vi "Periodic Tasks.vi"(8 "error in":errorcluster) -> ()   [LabVIEW 2019]
doc: "This VI runs in parallel to other tasks. It can contain as many user-defined periodic loops as you need. These can carry out PID or other sorts of timed response."
uses:
  <vilib>/Rock Robotics/WPI/DriverStation/WPI_DriverStationRobotMode2.ctl
  <vilib>/Rock Robotics/WPI/Utilities/WPI_GetSetVariantRefNum.vi
  Robot Global Data.vi
  <vilib>/Rock Robotics/WPI/RobotDrive/WPI_RobotDriveArcadeDrive_Standard(NoSaturation).vi
  <vilib>/Rock Robotics/Network Tables/NT Write Numeric Array.vi
  <vilib>/Rock Robotics/Network Tables/NT Write Number.vi
  <vilib>/Rock Robotics/Network Tables/NT Write String.vi
panel:
  in  "Yellow":cluster{"R":dbl, "G":dbl, "B":dbl}
  in  "Blue":cluster{"R":dbl, "G":dbl, "B":dbl}
  in  "Green":cluster{"R":dbl, "G":dbl, "B":dbl}
  in  "Red":cluster{"R":dbl, "G":dbl, "B":dbl}
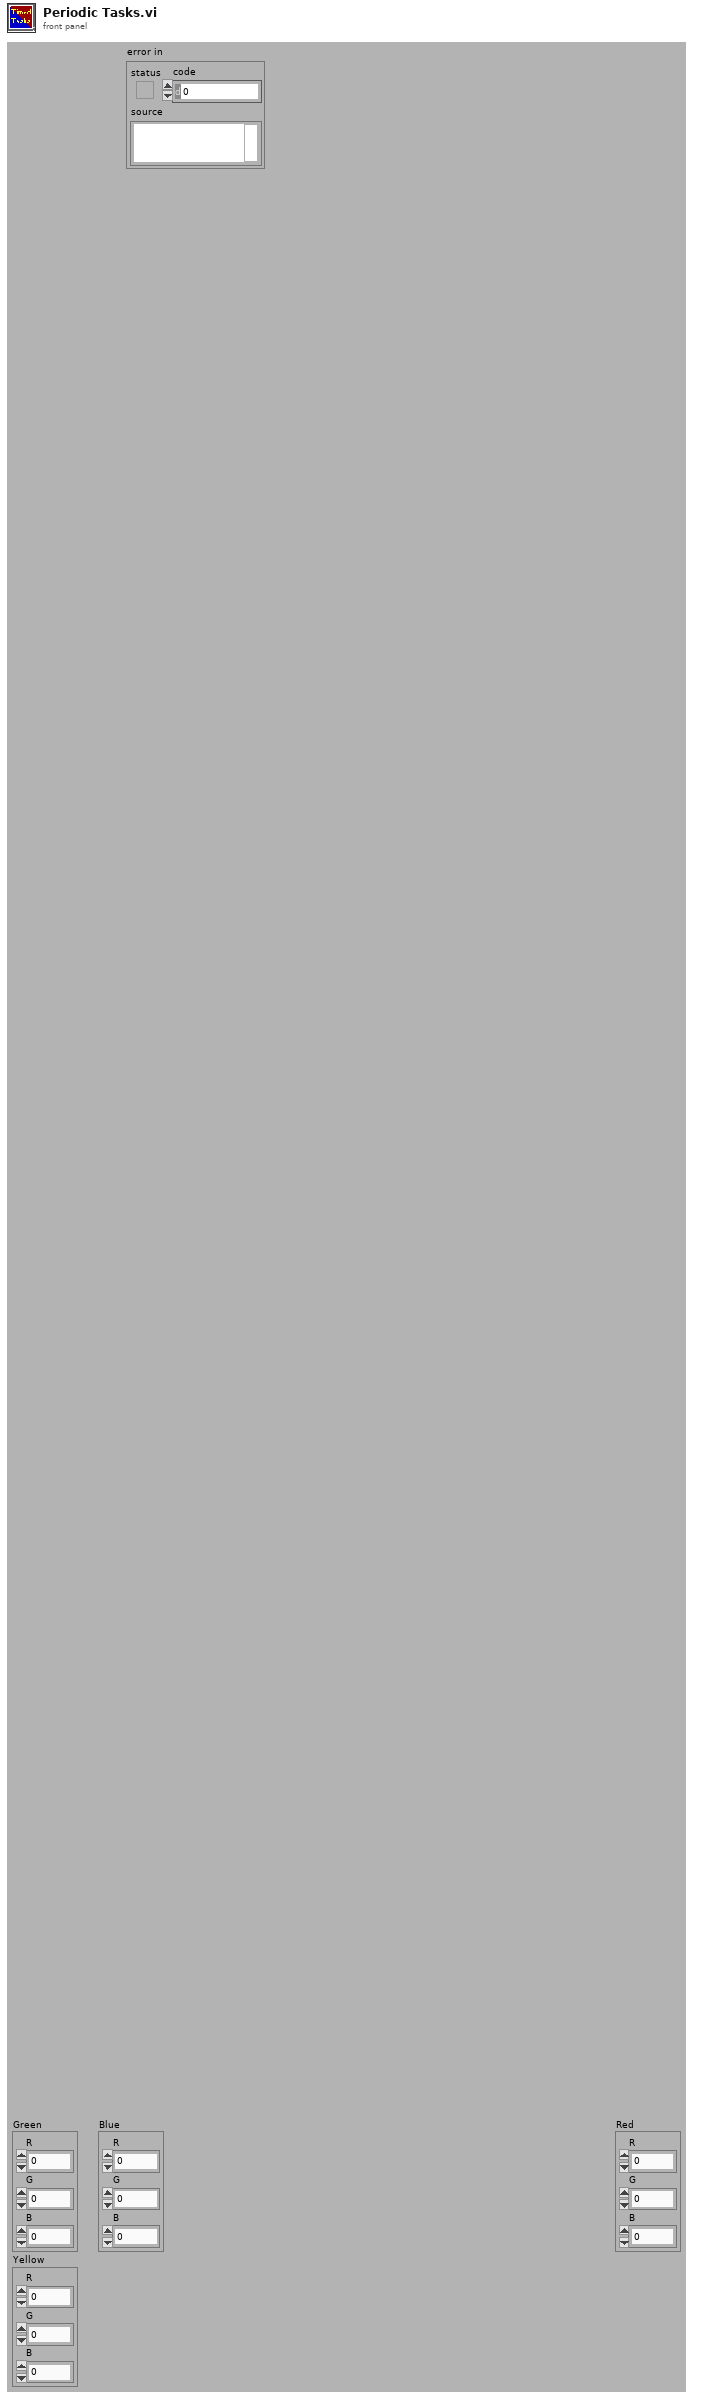
[diagram p1: front panel]
types:
  T1 = typedef "WPI_RobotDriveDevRef.ctl" = cluster{"DevStatus":errorcluster, "Motors[]":T2[], "Square Inputs":bool, "Max Output":dbl}
  T2 = typedef "WPI_MotorControlDeviceRef.ctl" = cluster{"DeviceStatus":errorcluster, "Type":T3, "PWM":cluster{"PWM Channel":T4, "DeadBand":T5}, "CAN":cluster{"Device Number":u8, "SetOutput VI Ref":variant, "GetOutput VI Ref":variant, "Enable VI Ref":variant, "Disable VI Ref":variant, "Data":variant}, "Invert":bool, "DIO PWM":cluster{"PWM \"Enable\" Channel":T4, "DIOChannel":T6, "PWM Rate":dbl}}
  T3 = typedef "WPI_MotorControlType.ctl" = enum16{"PWM", "CAN", "DIO PWM"}
  T4 = typedef "FPGA_DIOPWMChannel.ctl" = enum8{"PWM 0", "PWM 1", "PWM 2", "PWM 3", "PWM 4", "PWM 5", "PWM 6", "PWM 7", "PWM 8", "PWM 9", "PWM MXP 0", "PWM MXP 1", "PWM MXP 2", "PWM MXP 3", "PWM MXP 4", "PWM MXP 5", "PWM MXP 6", "PWM MXP 7", "PWM MXP 8", "PWM MXP 9", "Invalid"}
  T5 = typedef "WPI_PWMDeadband.ctl" = cluster{"Name":string, "maxPositivePwm":i32, "minPositivePwm":i32, "centerPwm":i32, "maxNegativePwm":i32, "minNegativePwm":i32, "angularRange":u16}
  T6 = typedef "FPGA_DIOChannel.ctl" = enum8{"DIO 0", "DIO 1", "DIO 2", "DIO 3", "DIO 4", "DIO 5", "DIO 6", "DIO 7", "DIO 8", "DIO 9", "DIO MXP 0", "DIO MXP 1", "DIO MXP 2", "DIO MXP 3", "DIO MXP 4", "DIO MXP 5", "DIO MXP 6", "DIO MXP 7", "DIO MXP 8", "DIO MXP 9", "DIO MXP 10", "DIO MXP 11", "DIO MXP 12", "DIO MXP 13", "DIO MXP 14", "DIO MXP 15", "SPI Port CS1", "SPI Port CS2", "SPI Port CS3", "SPI Port MISO", "SPI Port MOSI", "Invalid"}
  T7 = typedef "WPI_JoystickDevRef.ctl" = cluster{"Device":T8}
  T8 = typedef "WPI_JoystickDeviceEnum.ctl" = enum16{"USB 0", "USB 1", "USB 2", "USB 3", "USB 4", "USB 5"}
  T9 = cluster{"JoystickDevRef":T7, "RobotDriveDevRef":T1}
  T10 = typedef "WPI_DriverStationRobotMode2.ctl" = enum16{"Autonomous Disabled", "Autonomous Enabled", "Teleop Disabled", "Teleop Enabled", "Disconnected", "Finish", "Test Disabled", "Test Enabled", "Emergency Stopped"}
  T11 = typedef "Color Sensor V3 DevRef.ctl" = cluster{"I2CDevRef":T12}
  T12 = typedef "WPI_I2CDevRef.ctl" = cluster{"DevStatus":errorcluster, "Device Address":u8, "Handle":i32, "I2C Bus":T13}
  T13 = typedef "i2c_bus.ctl" = enum16{"I2C On-Board", "I2C MXP", "Invalid"}
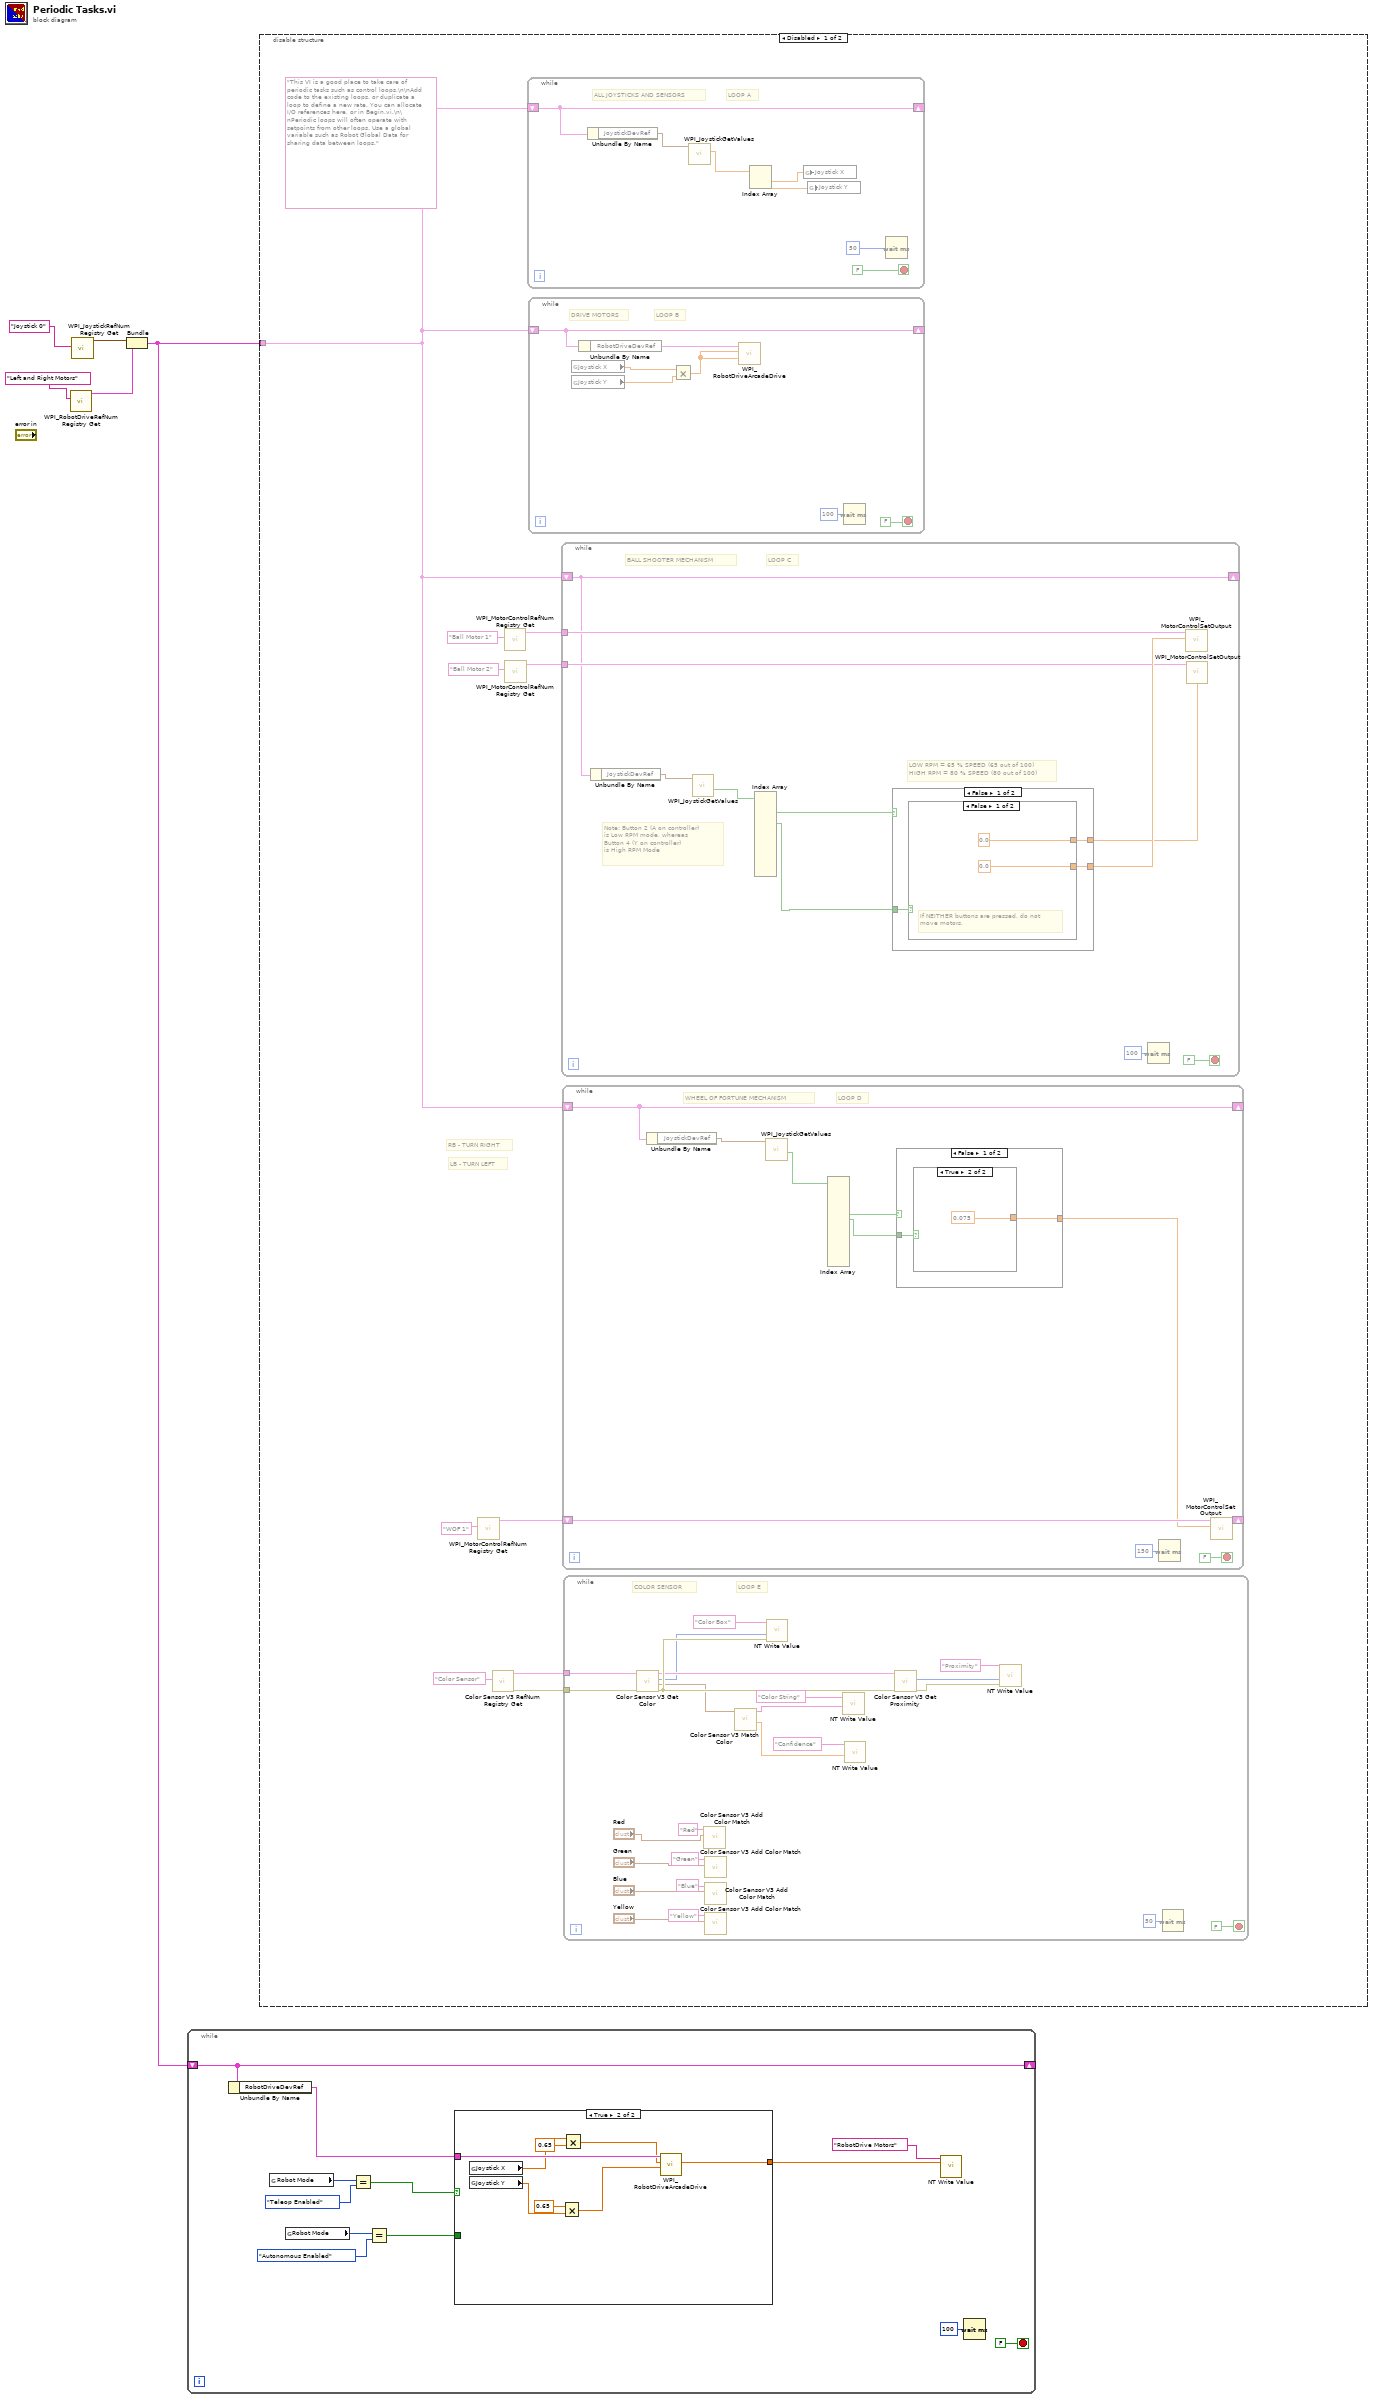
[diagram p0: block diagram]
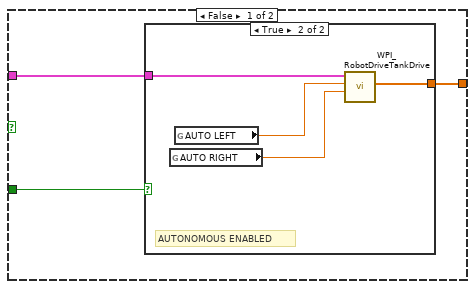
[diagram p2: hidden frame]
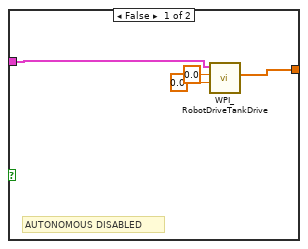
[diagram p3: hidden frame]
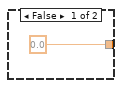
[diagram p4: hidden frame]
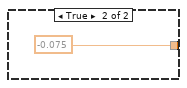
[diagram p5: hidden frame]
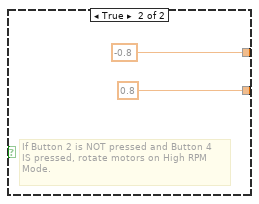
[diagram p6: hidden frame]
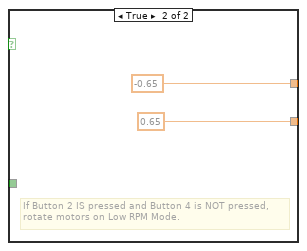
[diagram p7: hidden frame]
diagram:
  n1 = call <vilib>:"WPI_RobotDriveRefNum Registry Get.vi"("refnum name"="Left and Right Motors") -> ("RobotDriveDevRef"=w5:T1)  [unwired: 1 in, 9 out]
  n2 = call <vilib>:"WPI_JoystickRefNum Registry Get.vi"("refnum name"="Joystick 0") -> ("JoystickDevRef"=w4:T7)  [unwired: 1 in, 9 out]
  n3 = Bundle("JoystickDevRef"=w4, "RobotDriveDevRef"=w5) -> (w1:T9)  [unwired: 1 out]
  n4 = while {
    shift-right: [w17] -> _
    shift-left: w1 -> [w17]
    stop <- FALSE stop-if-true
    n5 = Unbundle By Name(w17) -> ("RobotDriveDevRef"=w12:T1)
    n6 = global read "Robot Global Data.vi" "Robot Mode"() -> (w10:T10)
    n7 = global read "Robot Global Data.vi" "Robot Mode"() -> (w8:T10)
    n8 = Equal?(x=w10, y=WPI_DriverStationRobotMode2."Teleop Enabled") -> (x = y?=w11:bool)
    n9 = Equal?(x=w8, y=WPI_DriverStationRobotMode2."Autonomous Enabled") -> (x = y?=w6:bool)
    n10 = case shown="True" w11 {
      tunnel: [w20 w35] -> w13
      tunnel: w12 -> [w19 w36]
      tunnel: w6 -> [w18 _]
      frame False {
        n11 = case shown="True" w18 {
          tunnel: [w24 w28] -> w20
          tunnel: w19 -> [w21 w26]
          frame False {
            # "AUTONOMOUS DISABLED"
            n12 = call <vilib>:"WPI_RobotDriveTankDrive.vi"("Right axis value"=0.0, "Left axis value"=0.0, "RobotDriveDevRef"=w21) -> ("Motor Values"=w24:dbl[])  [unwired: 6 in, 2 out]
          }
          frame True {
            # "AUTONOMOUS ENABLED"
            n13 = global read "Robot Global Data.vi" "AUTO RIGHT"() -> (w25:dbl)
            n14 = global read "Robot Global Data.vi" "AUTO LEFT"() -> (w27:dbl)
            n15 = call <vilib>:"WPI_RobotDriveTankDrive.vi"("Right axis value"=w25, "Left axis value"=w27, "RobotDriveDevRef"=w26) -> ("Motor Values"=w28:dbl[])  [unwired: 6 in, 2 out]
          }
        }
      }
      frame True {
        n16 = global read "Robot Global Data.vi" "Joystick X"() -> (w34:dbl)
        n17 = global read "Robot Global Data.vi" "Joystick Y"() -> (w33:dbl)
        n18 = Multiply(x=0.65, y=w33) -> (x*y=w29:dbl)
        n19 = Multiply(x=w34, y=0.65) -> (x*y=w30:dbl)
        n20 = call-poly <vilib>:"WPI_RobotDriveArcadeDrive.vi"("Y axis value"=w29, "X axis value"=w30, "RobotDriveDevRef"=w36) -> ("Motor Values"=w35:dbl[])  [unwired: 6 in, 2 out]
      }
    }
    n21 = call-poly <vilib>:"NT Write Value.vi"("Numeric Array"=w13, "Name"="RobotDrive Motors") -> ()  [unwired: 9 in, 1 out]
    n22 = Wait (ms)(milliseconds to wait=u32 100) -> ()  [unwired: 1 out]
  }
  n23 = disable-structure shown="Disabled" {
    disable-tunnel: w1 -> [w37 _]
    frame Disabled {
      (unwired) "This VI is a good place to take care of periodic tasks such as control loops.\n\nAdd code to the existing loops, or duplicate a loop to define a new rate. You can allocate I/O references here, or in Begin.vi.\n\nPeriodic loops will often operate with setpoints from other loops. Use a global variable such as Robot Global Data for sharing data between loops."
      # "LB - TURN LEFT"
      # "RB - TURN RIGHT"
      n24 = call <vilib>:"WPI_MotorControlRefNum Registry Get.vi"("refnum name"="WOF 1") -> ("MotorControlDevRef"=w41:T2)  [unwired: 9 in, 1 out]
      n25 = call <vilib>:"Color Sensor V3 RefNum Registry Get.vi"("refnum name"="Color Sensor") -> ("error out"=w38:errorcluster, "ColorSensorDevRef"=w40:T11)  [unwired: 9 in]
      n26 = call <vilib>:"WPI_MotorControlRefNum Registry Get.vi"("refnum name"="Ball Motor 1") -> ("MotorControlDevRef"=w44:T2)  [unwired: 9 in, 1 out]
      n27 = call <vilib>:"WPI_MotorControlRefNum Registry Get.vi"("refnum name"="Ball Motor 2") -> ("MotorControlDevRef"=w43:T2)  [unwired: 9 in, 1 out]
      n28 = while {
        shift-right: [w118] -> _
        shift-left: w37 -> [w118]
        stop <- FALSE stop-if-true
        # "LOOP A"
        # "ALL JOYSTICKS AND SENSORS"
        n29 = Unbundle By Name(w118) -> ("JoystickDevRef"=w117:T7)
        n30 = call <vilib>:"WPI_JoystickGetValues.vi"("JoystickDevRef"=w117) -> ("Axes"=w116:dbl[])  [unwired: 6 in, 4 out]
        n31 = Index Array(array=w116) -> (element #1=w114:dbl, element #2=w115:dbl)  [unwired: 2 in]
        n32 = global write "Robot Global Data.vi" "Joystick X"(w114) -> ()
        n33 = global write "Robot Global Data.vi" "Joystick Y"(w115) -> ()
        n34 = Wait (ms)(milliseconds to wait=u32 50) -> ()  [unwired: 1 out]
      }
      n35 = while {
        shift-right: [w110] -> _
        shift-left: w37 -> [w110]
        stop <- FALSE stop-if-true
        # "LOOP B"
        # "DRIVE MOTORS"
        n36 = global read "Robot Global Data.vi" "Joystick X"() -> (w106:dbl)
        n37 = global read "Robot Global Data.vi" "Joystick Y"() -> (w107:dbl)
        n38 = Unbundle By Name(w110) -> ("RobotDriveDevRef"=w109:T1)
        n39 = Multiply(x=w106, y=w107) -> (x*y=w108:dbl)
        n40 = call-poly <vilib>:"WPI_RobotDriveArcadeDrive.vi"("Y axis value"=w108, "X axis value"=w108, "RobotDriveDevRef"=w109) -> ()  [unwired: 6 in, 3 out]
        n41 = Wait (ms)(milliseconds to wait=u32 100) -> ()  [unwired: 1 out]
      }
      n42 = while {
        shift-right: [w90] -> _
        shift-left: w37 -> [w90]
        tunnel: w44 -> [w94]
        tunnel: w43 -> [w91]
        stop <- FALSE stop-if-true
        # "LOW RPM = 65 % SPEED (65 out of 100)\nHIGH RPM = 80 % SPEED (80 out of 100)"
        # "LOOP C"
        # "Note: Button 2 (A on controller) \nis Low RPM mode, whereas \nButton 4 (Y on controller)\nis High RPM Mode"
        # "BALL SHOOTER MECHANISM"
        n43 = Unbundle By Name(w90) -> ("JoystickDevRef"=w89:T7)
        n44 = call <vilib>:"WPI_JoystickGetValues.vi"("JoystickDevRef"=w89) -> ("Buttons"=w88:bool[])  [unwired: 6 in, 4 out]
        n45 = Index Array(array=w88) -> (element #2=w86:bool, element #4=w87:bool)  [unwired: 13 in, 11 out]
        n46 = case shown="False" w86 {
          tunnel: [w99 0.65 ("Output")] -> w93
          tunnel: [w98 -0.65 ("Output")] -> w92
          tunnel: w87 -> [w97 _]
          frame False {
            n47 = case shown="False" w97 {
              tunnel: [0.0 ("Output") 0.8 ("Output")] -> w99
              tunnel: [0.0 ("Output") -0.8 ("Output")] -> w98
              frame False {
                # "If NEITHER buttons are pressed, do not\nmove motors."
              }
              frame True {
                # "If Button 2 is NOT pressed and Button 4\nIS pressed, rotate motors on High RPM\nMode."
              }
            }
          }
          frame True {
            # "If Button 2 IS pressed and Button 4 is NOT pressed,\nrotate motors on Low RPM Mode."
          }
        }
        n48 = Wait (ms)(milliseconds to wait=u32 100) -> ()  [unwired: 1 out]
        n49 = call <vilib>:"WPI_MotorControlSetOutput.vi"("Output"=w93, "MotorControlDevRef"=w94) -> ()  [unwired: 7 in, 3 out]
        n50 = call <vilib>:"WPI_MotorControlSetOutput.vi"("Output"=w92, "MotorControlDevRef"=w91) -> ()  [unwired: 7 in, 3 out]
      }
      n51 = while {
        shift-right: [w79] -> _
        shift-left: w37 -> [w79]
        shift-right: [w75] -> _
        shift-left: w41 -> [w76]
        stop <- FALSE stop-if-true
        # "LOOP D"
        # "WHEEL OF FORTUNE MECHANISM"
        n52 = Unbundle By Name(w79) -> ("JoystickDevRef"=w78:T7)
        n53 = call <vilib>:"WPI_JoystickGetValues.vi"("JoystickDevRef"=w78) -> ("Buttons"=w77:bool[])  [unwired: 6 in, 4 out]
        n54 = Index Array(array=w77) -> (element #5=w73:bool, element #6=w72:bool)  [unwired: 14 in, 12 out]
        n55 = case shown="False" w73 {
          tunnel: [w81 -0.075 ("Output")] -> w74
          tunnel: w72 -> [w82 _]
          frame False {
            n56 = case shown="True" w82 {
              tunnel: [0.0 ("Output") 0.075 ("Output")] -> w81
              frame False {
              }
              frame True {
              }
            }
          }
          frame True {
          }
        }
        n57 = Wait (ms)(milliseconds to wait=u32 150) -> ()  [unwired: 1 out]
        n58 = call <vilib>:"WPI_MotorControlSetOutput.vi"("Output"=w74, "MotorControlDevRef"=w76) -> ("MotorControlDevRef"=w75:T2)  [unwired: 7 in, 2 out]
      }
      n59 = while {
        tunnel: w40 -> [w69]
        tunnel: w38 -> [w68]
        stop <- FALSE stop-if-true
        # "LOOP E"
        # "COLOR SENSOR"
        n60 = call <vilib>:"Color Sensor V3 Get Color.vi"("error in (no error)"=w68, "ColorSensorDevRef"=w69) -> ("error out"=w67:errorcluster, "Normalized Color"=w61:cluster{"R":dbl, "G":dbl, "B":dbl}, "Color"=w64:u32, "ColorSensorDevRef out"=w65:T11)  [unwired: 6 in]
        n61 = call <vilib>:"Color Sensor V3 Add Color Match.vi"("Color"="Red", "Name"="Red") -> ()  [unwired: 10 in]
        n62 = call <vilib>:"Color Sensor V3 Add Color Match.vi"("Color"="Green", "Name"="Green") -> ()  [unwired: 10 in]
        n63 = call <vilib>:"Color Sensor V3 Add Color Match.vi"("Color"="Blue", "Name"="Blue") -> ()  [unwired: 10 in]
        n64 = call <vilib>:"Color Sensor V3 Add Color Match.vi"("Color"="Yellow", "Name"="Yellow") -> ()  [unwired: 10 in]
        n65 = call <vilib>:"Color Sensor V3 Match Color.vi"("Measured Color"=w61) -> ("Confidence"=w60:dbl, "Matched Color Name"=w59:string)  [unwired: 8 in, 1 out]
        n66 = call-poly <vilib>:"NT Write Value.vi"("error in"=w67, "Numeric"=w64, "Name"="Color Box") -> ()  [unwired: 8 in, 1 out]
        n67 = call-poly <vilib>:"NT Write Value.vi"("String"=w59, "Name"="Color String") -> ()  [unwired: 9 in, 1 out]
        n68 = call-poly <vilib>:"NT Write Value.vi"("Numeric"=w60, "Name"="Confidence") -> ()  [unwired: 9 in, 1 out]
        n69 = call <vilib>:"Color Sensor V3 Get Proximity.vi"("error in (no error)"=w67, "ColorSensorDevRef"=w65) -> ("error out"=w62:errorcluster, "Proximity"=w63:u16)  [unwired: 7 in, 1 out]
        n70 = call-poly <vilib>:"NT Write Value.vi"("error in"=w62, "Numeric"=w63, "Name"="Proximity") -> ()  [unwired: 8 in, 1 out]
        n71 = Wait (ms)(milliseconds to wait=u32 50) -> ()  [unwired: 1 out]
      }
    }
    frame Enabled {
    }
  }
